vi "SSL Vision Package Selector.vi"(7 "timeout in ms (-1)":i32=-1, 9 "channel in":T2, 10 "Channel in":T1, 11 "Modo":bool) -> (3 "element":u8[](array[numeric]))   [LabVIEW 2016]
uses:
  <extravilib>/ChannelInstances/Stream-a[.](u8)/)Channel.ctl
  <extravilib>/ChannelInstances/Lossy Stream-a[.](u8)/)Channel.ctl
  <extravilib>/ChannelInstances/Stream-a[.](u8)/Read With Abort.vi
  <extravilib>/ChannelInstances/Lossy Stream-a[.](u8)/Read With Abort.vi
  <extravilib>/ChannelInstances/Stream-a[.](u8)/Endpoint.vi
  <extravilib>/ChannelInstances/Lossy Stream-a[.](u8)/Endpoint.vi
  <extravilib>/ChannelInstances/Stream-a[.](u8)/)Channel.vi
  <resource>/ChannelSupport/_ChannelSupport/WaitIfNeeded.vi
  <extravilib>/ChannelInstances/Lossy Stream-a[.](u8)/)Channel.vi
  <extravilib>/ChannelInstances/Lossy Stream-a[.](u8).lvlib
  <extravilib>/ChannelInstances/Stream-a[.](u8).lvlib
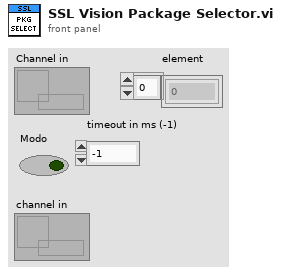
[diagram p1: front panel]
types:
  T1 = typedef "Lossy Stream-a[.](u8).lvlib/)Channel.ctl" = refnum<queue>
  T2 = typedef "Stream-a[.](u8).lvlib/)Channel.ctl" = refnum<queue>
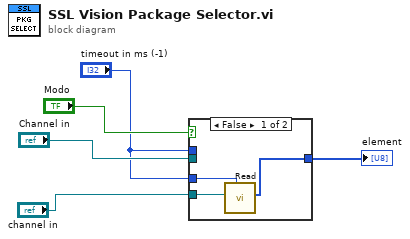
[diagram p0: block diagram]
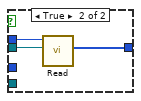
[diagram p2: hidden frame]
diagram:
  n1 = case shown="False" "Modo" {
    tunnel: [w7 w11] -> w4
    tunnel: "channel in" -> [w8 _]
    tunnel: "timeout in ms (-1)" -> [w6 _]
    tunnel: "Channel in" -> [_ w10]
    tunnel: "timeout in ms (-1)" -> [_ w9]
    frame False {
      n2 = call <extravilib>:"Read.vi"("timeout in ms (-1)"=w6, "channel"=w8) -> ("element"=w7:u8[])  [unwired: 5 in, 4 out]
    }
    frame True {
      n3 = call <extravilib>:"Read.vi"("channel"=w10, "timeout in ms (-1)"=w9) -> ("element"=w11:u8[])  [unwired: 4 in, 5 out]
    }
  }
  "element" <- w4
